vi "Read Send Header String.vi"(8 "error in (no error)":errorcluster, 11 "WebSocket in":refnum<class "WebSocket.lvclass">) -> (0 "error out":errorcluster, 2 "Send Header String":string, 3 "WebSocket out":refnum<class "WebSocket.lvclass">)   [LabVIEW 2021, in "WebSockets.lvlib" / "WebSocket.lvclass"]
doc: "Generates HTTP header string from the send headers.\nWebSockets 2.0.1.40\nSam Sharp - MediaMongrels Ltd\nCopyright (c) 2019, MediaMongrels Ltd"
uses:
  WebSocket.lvclass
  WebSocket.lvclass/WebSocket.ctl
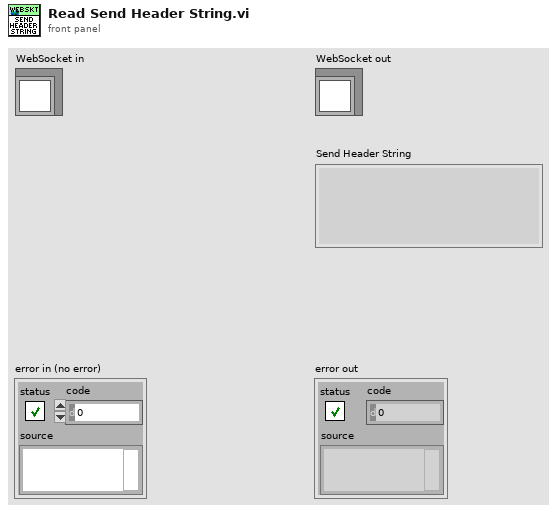
[diagram p1: front panel]
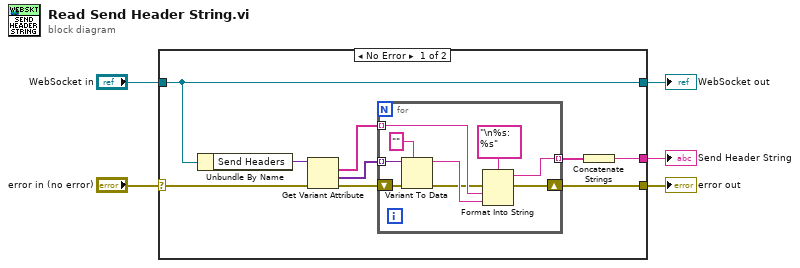
[diagram p0: block diagram]
diagram:
  n1 = case shown="No Error" "error in (no error)" {
    selector: "error in (no error)" -> [w10 w25]
    tunnel: [w6 w25] -> w4
    tunnel: [w14 w24] -> w2
    tunnel: "WebSocket in" -> [w14 w24]
    tunnel: [w8 _] -> w1
    frame No Error {
      n2 = Unbundle By Name(w14) -> ("Send Headers"=w13:variant)
      n3 = Get Variant Attribute(Variant=w13, error in=w10) -> (names=w12:string[], values=w11:variant[], error out=w7:errorcluster)  [unwired: 2 in, 1 out]
      n4 = for {
        tunnel: w12 -> [w22] mode=indexing
        tunnel: w11 -> [w17] mode=indexing
        tunnel: [w21] -> w9 mode=indexing
        shift-right: [w15] -> w6
        shift-left: w7 -> [w20]
        n5 = Variant To Data(error in=w20, type="", Variant=w17) -> (data=w19:string, error out=w18:errorcluster)
        n6 = Format Into String(format string="\n%s: %s", error in=w18, w22, w19) -> (resulting string=w21:string, error out=w15:errorcluster)  [unwired: 1 in]
      }
      n7 = Concatenate Strings(w9) -> (w8:string)
    }
    frame Error {
    }
  }
  "error out" <- w4
  "WebSocket out" <- w2
  "Send Header String" <- w1
